vi "SetWindowHitTest.vi"(8 "No Error":errorcluster, 9 "Data [void *]":i64 format="%.0x", 10 "Callback [(*SDL_HitTest)]":i64 format="%.0x", 11 "Window [SDL_Window *]":i64 format="%.0x") -> (0 "Error Out":errorcluster)   [LabVIEW 2024, in "SDL3.lvlib" / "Video.lvlib"]
doc: "<B>Summary</B>\nProvide a callback that decides if a window region has special properties.\n\n<B>Remarks</B>\nNormally windows are dragged and resized by decorations provided by the system window manager (a title bar, borders, etc), but for some apps, it makes sense to drag them from somewhere else inside the window itself; for example, one might have a borderless window that wants to be draggable from any part, or simulate its own title bar, etc.\n\nThis function lets the app provide a callback that designates pieces of a given window as special. This callback is run during event processing if we need to tell the OS to treat a region of the window specially; the use of this callback is known as \"hit testing.\"\n\nMouse input may not be delivered to your application if it is within a special area; the OS will often apply that input to moving the window or resizing the window and not deliver it to the application.\n\nSpecifying NULL for a callback disables hit-testing. Hit-testing is disabled by default.\n\nPlatforms that don't support this functionality will return false unconditionally, even if you're attempting to disable hit-testing.\n\nYour callback may fire at any time, and its firing does not indicate any specific behavior (for example, on Windows, this certainly might fire when the OS is deciding whether to drag your window, but it fires for lots of other reasons, too, some unrelated to anything you probably care about and when the mouse isn't actually at the location it is testing). Since this can fire at any time, you should try to keep your callback efficient, devoid of allocations, etc."
uses:
  Video.lvlib
  Lib/SDL3.dll
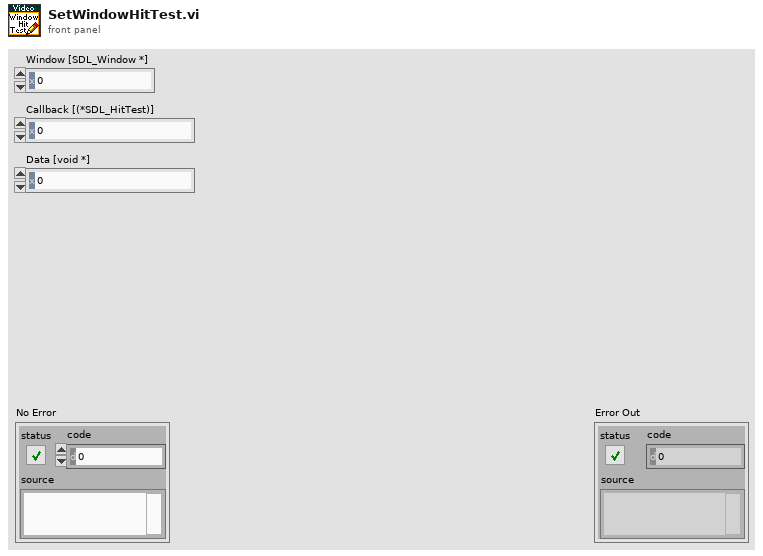
[diagram p1: front panel]
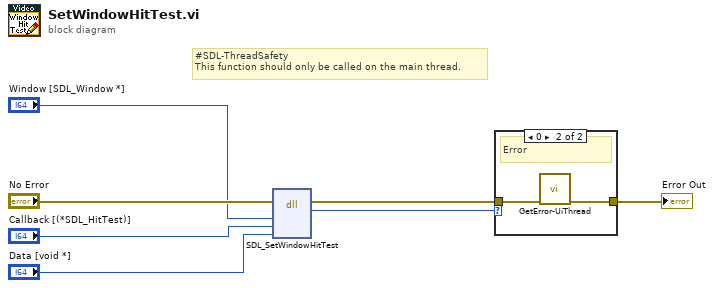
[diagram p0: block diagram]
diagram:
  # "#SDL-ThreadSafety\nThis function should only be called on the main thread."
  n1 = dll-call lib="C:/Users/Thomas/Documents/Projects/LV-SDL3/Sources/SDL3/Lib/SDL3.*" fn="SDL_SetWindowHitTest"(error in="No Error", "window"="Window [SDL_Window *]", "callback"="Callback [(*SDL_HitTest)]", "callback_data"="Data [void *]") -> (error out=w4:errorcluster, "return type"=w3:i32)  [unwired: 5 in, 1 out]
  n2 = case shown="0" w3 {
    tunnel: w4 -> [w8 w10]
    tunnel: [w8 w9] -> w6
    frame Default {
      # "Ok"
    }
    frame 0 {
      # "Error"
      n3 = call "GetError-UiThread.vi"("No Error"=w10) -> ("error out"=w9:errorcluster)  [unwired: 10 in]
    }
  }
  "Error Out" <- w6
